vi "DHT (2).vi"() -> ()   [LabVIEW 2017]
uses:
  <vilib>/MakerHub/LINX/Public/Utilities/Open Serial.vi
  <vilib>/MakerHub/LINX/LMH-LINX.lvlib
panel:
  in  "Serial Port":refnum<visa-resource-name>="N/A"
  out "CHAUD":bool
  out "FROID":bool
  out "Statut de Temperature":string
  out "NORMAL":bool
  in  "MIN":dbl
  in  "MAX":dbl
  out "Temperature en °C":u8(knob) scale=0.0..50.0
  out "Humidité en %":u8(knob) scale=0.0..100.0
  in  "?":bool
  # "Aquisition de la température et l'humidité en utilisant Arduino, LabVIEW et capteur DHT11"
  # "DHT11"
  # "Ce projet est réalisé par : INNAN Nouhaila          Encadré par Professeur:S.OUASKIT"
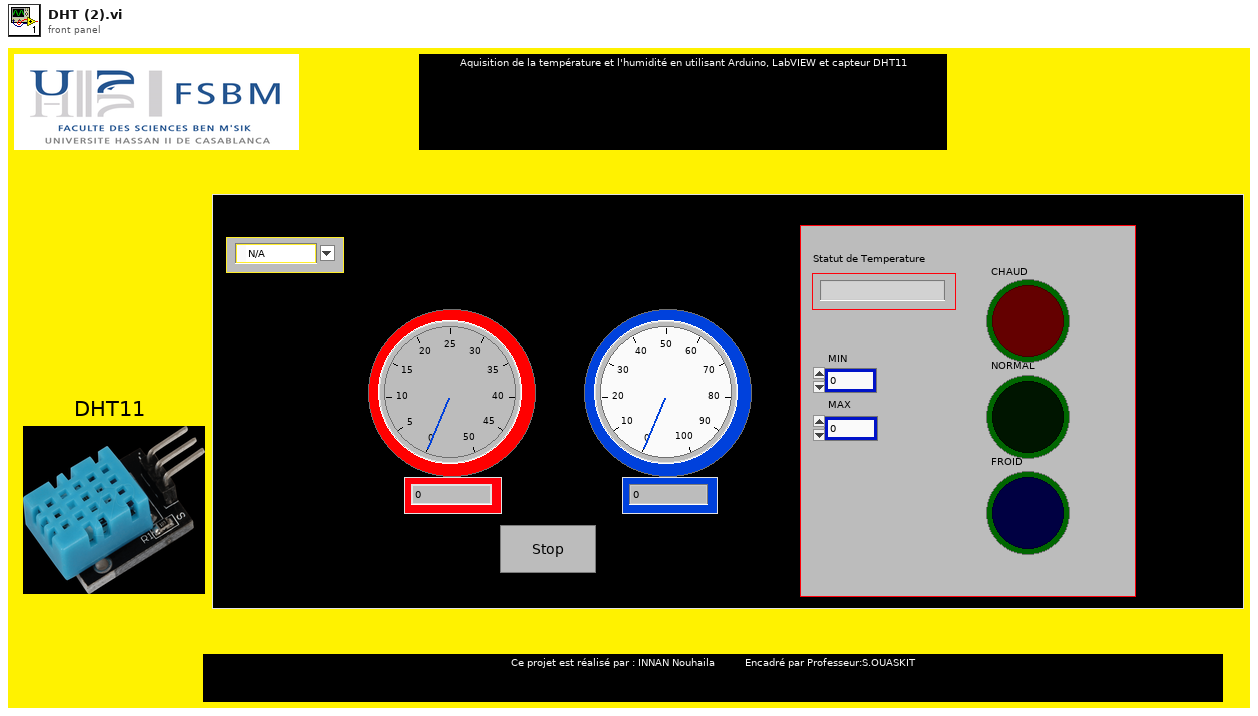
[diagram p1: front panel]
types:
  T1 = typedef "LMH-LINX.lvlib/LINX Ref.ctl" = cluster{"IO":T2, "Interface":T3, "LINX Device Config":T4}
  T2 = typedef "LMH-LINX.lvlib/Platform.ctl" = enum16{"Remote", "Local"}
  T3 = typedef "LMH-LINX.lvlib/Interface.ctl" = enum16{"Serial", "TCP"}
  T4 = typedef "LMH-LINX.lvlib/Device.lvlib/LINX Device Config.ctl" = cluster{"Interface":T3, "COM Port":refnum<visa-resource-name>, "TCP Configuration":T5, "Device Family":u8, "Device ID":u8, "Device Name":string, "TCP Ref":refnum<k5>, "Channels":T6}
  T5 = typedef "LMH-LINX.lvlib/Device.lvlib/TCP Config.ctl" = cluster{"IP Address":string, "Port":u16}
  T6 = typedef "LMH-LINX.lvlib/Channels.ctl" = cluster{"DI":u8[], "DO":u8[], "AI":u8[], "AO":u8[], "PWM":u8[], "QE":u8[], "UART":u8[], "I2C 2":u8[], "SPI":u8[], "CAN":u8[], "Servo":u8[], "AI Ref (V)":dbl, "AI Resolution (Bits)":u8, "AO Ref (V)":dbl, "AO Resolution (Bits)":u8}
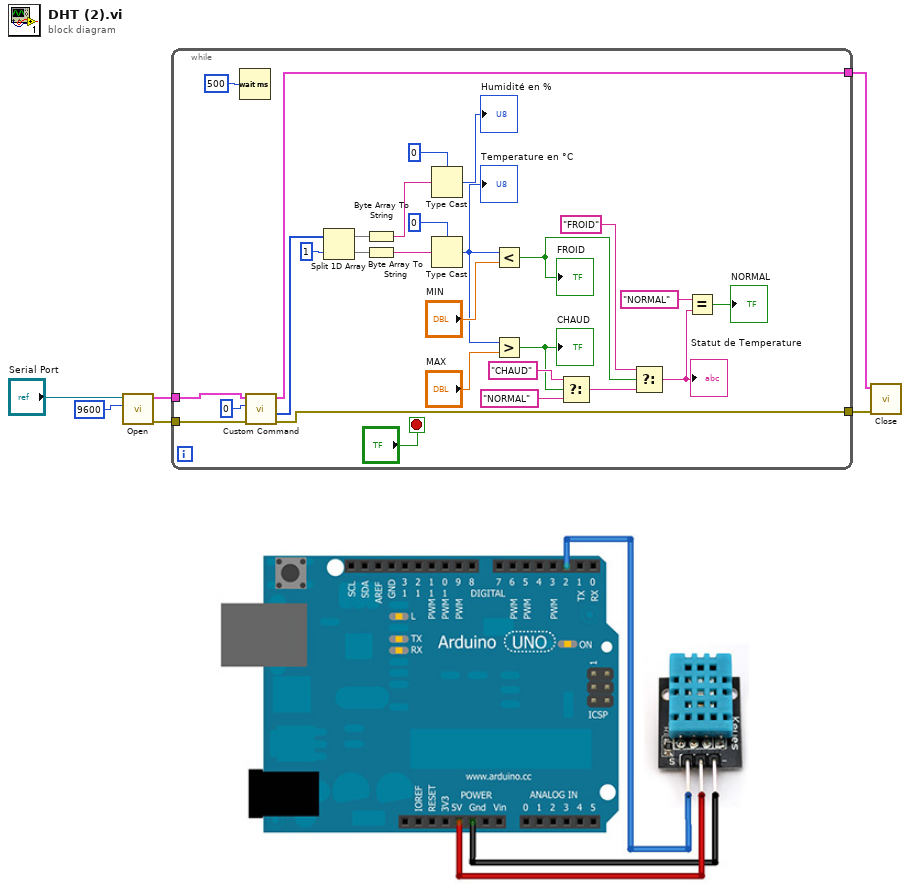
[diagram p0: block diagram]
diagram:
  n1 = call-poly <vilib>:"Open.vi"("Baud Rate Override"=u32 9600, "Serial Port"="Serial Port") -> ("Error Out"=w5:errorcluster, "LINX Resource"=w6:T1)  [unwired: 7 in, 1 out]
  n2 = while {
    tunnel: w6 -> [w34]
    tunnel: w5 -> [w33]
    tunnel: [w32] -> w4
    tunnel: [w8] -> w3
    stop <- "?" stop-if-true
    n3 = Wait (ms)(milliseconds to wait=u32 500) -> ()  [unwired: 1 out]
    n4 = call <vilib>:"Custom Command.vi"("Error In"=w33, "Custom Command Number"=u16 0, "LINX Resource"=w34) -> ("Error Out"=w8:errorcluster, "Response"=w29:u8[], "LINX Resource"=w32:T1)  [unwired: 5 in, 1 out]
    n5 = Split 1D Array(array=w29, index=1) -> (first subarray=w27:u8[], second subarray=w26:u8[])
    n6 = Byte Array To String(unsigned byte array=w27) -> (string=w24:string)
    n7 = Byte Array To String(unsigned byte array=w26) -> (string=w22:string)
    n8 = Type Cast(type=u8 0, x=w24) -> (*(type *) &x=→"Humidité en %":u8)
    n9 = Type Cast(type=u8 0, x=w22) -> (*(type *) &x=w9:u8)
    "Temperature en °C" <- w9
    n10 = Less?(x=w9, y="MIN") -> (x < y?=w13:bool)
    "FROID" <- w13
    n11 = Greater?(x=w9, y="MAX") -> (0:w11:bool)
    "CHAUD" <- w11
    n12 = Select(t="CHAUD", s=w11, f="NORMAL") -> (s? t:f=w16:string)
    n13 = Select(t="FROID", s=w13, f=w16) -> (s? t:f=w14:string)
    "Statut de Temperature" <- w14
    n14 = Equal?(x="NORMAL", y=w14) -> (x = y?=→"NORMAL":bool)
  }
  n15 = call <vilib>:"Close.vi"("Error In"=w3, "LINX Resource"=w4) -> ()  [unwired: 9 in, 1 out]
